vi "$ICXX.vi"(11 "反馈信息":string) -> (3 "接收信息":T1)   [LabVIEW 2016, in "环境动力监测库.lvlib" / "NMEA.lvlib"]
uses:
  NMEA.lvlib
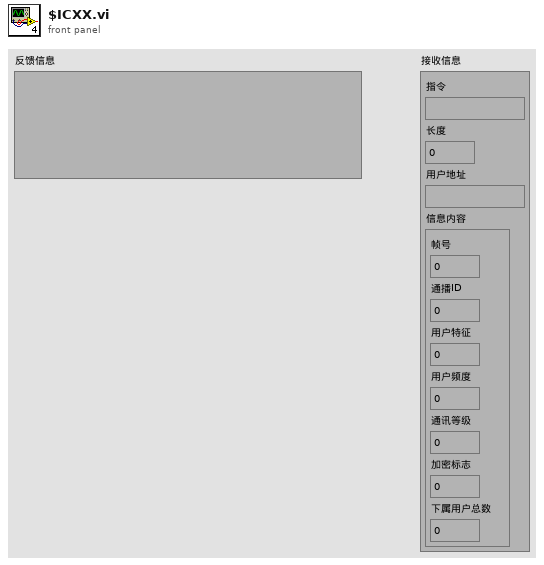
[diagram p1: front panel]
types:
  T1 = cluster{"指令":string, "长度":u16, "用户地址":string, "信息内容":cluster{"帧号":u8, "通播ID":u32, "用户特征":u8, "用户频度":u16, "通讯等级":u8, "加密标志":u8, "下属用户总数":u16}}
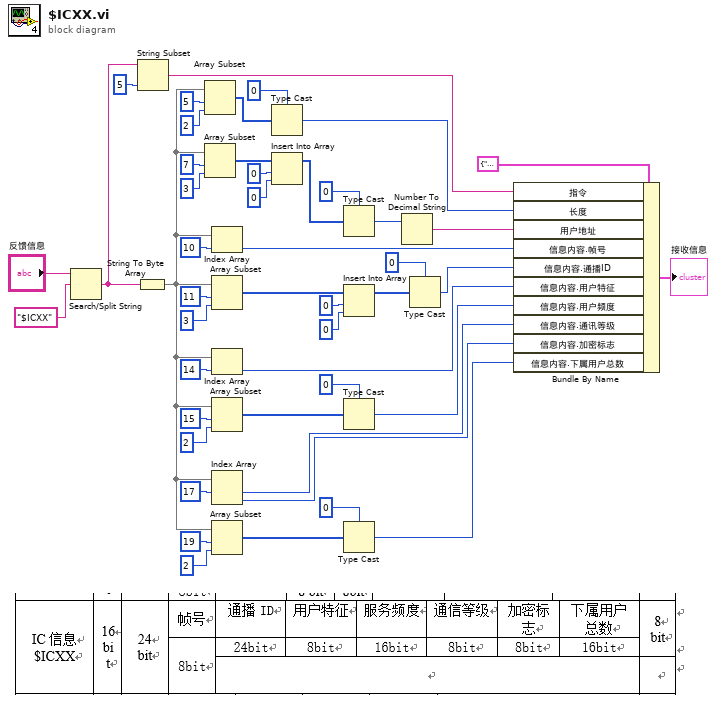
[diagram p0: block diagram]
diagram:
  n1 = Search/Split String(string="反馈信息", search string/char (-)="$ICXX" ("搜索字符串/字符(-)")) -> (match + rest of string=w45:string)  [unwired: 1 in, 2 out]
  n2 = String To Byte Array(string=w45) -> (unsigned byte array=w16:u8[])
  n3 = String Subset(string=w45, length (rest)=5 ("长度（剩余）")) -> (substring=w43:string)  [unwired: 1 in]
  n4 = Array Subset(array=w16, index=5 ("索引"), length=2 ("长度")) -> (w40:u8[])
  n5 = Array Subset(array=w16, index=7 ("索引"), length=3 ("长度")) -> (w10:u8[])
  n6 = Index Array(array=w16, index=10 ("索引")) -> (element=w34:u8)
  n7 = Array Subset(array=w16, index=11 ("索引"), length=3 ("长度")) -> (w28:u8[])
  n8 = Index Array(array=w16, index=14 ("索引")) -> (element=w25:u8)
  n9 = Array Subset(array=w16, index=15 ("索引"), length=2 ("长度")) -> (w22:u8[])
  n10 = Index Array(array=w16, index #1=17 ("索引")) -> (element #1=w18:u8, element #2=w17:u8)  [unwired: 1 in]
  n11 = Array Subset(array=w16, index=19 ("索引"), length=2 ("长度")) -> (w13:u8[])
  n12 = Type Cast(type=u16 0 ("长度"), x=w40) -> (*(type *) &x=w38:u16)
  n13 = Insert Into Array(array=w10, index=0 ("索引"), new element=u8 0 ("新元素/子数组")) -> (w6:u8[])
  n14 = Type Cast(type=u32 0 ("长度"), x=w6) -> (*(type *) &x=w8:u32)
  n15 = Insert Into Array(array=w28, index=0 ("索引"), new element=u8 0 ("新元素/子数组")) -> (w3:u8[])
  n16 = Type Cast(type=u16 0, x=w22) -> (*(type *) &x=w20:u16)
  n17 = Type Cast(type=u16 0, x=w13) -> (*(type *) &x=w11:u16)
  n18 = Number To Decimal String(number=w8) -> (decimal integer string=w7:string)  [unwired: 1 in]
  n19 = Type Cast(type=0, x=w3) -> (*(type *) &x=w27:i32)
  n20 = Bundle By Name(cluster=T1 {"指令"="", "长度"=0, "用户地址"="", "信息内容"={"帧号"=0, "通播ID"=0, "用户特征"=0, "用户频度"=0, "通讯等级"=0, "加密标志"=0, "下属用户总数"=0}} ("接收信息"), "指令"=w43, "长度"=w38, "用户地址"=w7, "信息内容.帧号"=w34, "信息内容.通播ID"=w27, "信息内容.用户特征"=w25, "信息内容.用户频度"=w20, "信息内容.通讯等级"=w18, "信息内容.加密标志"=w17, "信息内容.下属用户总数"=w11) -> (→"接收信息":T1)
